vi "Error Process.vi"(8 "error in (no error)":errorcluster, 11 "View Model":T1) -> (0 "error out":errorcluster)   [LabVIEW 2017]
doc: "The Elevator has centralized error handling with three categories of errors."
uses:
  View Model/Controls/View Model.ctl
  View Model/Controls/Shared Model.ctl
  Controls/Error Model.ctl
  Controls/Error Event.ctl
  Controls/Error Type.ctl
  Configuration/Controls/Config DB Model.ctl
  Configuration/Controls/Config DB Command.ctl
  Configuration/Controls/Config DB Record.ctl
  Controller/Controls/Controller Model.ctl
  Controller/Controls/Elevator Location.ctl
  Controller/Controls/Elevator Direction Event.ctl
  Controller/Controls/Elevator Direction.ctl
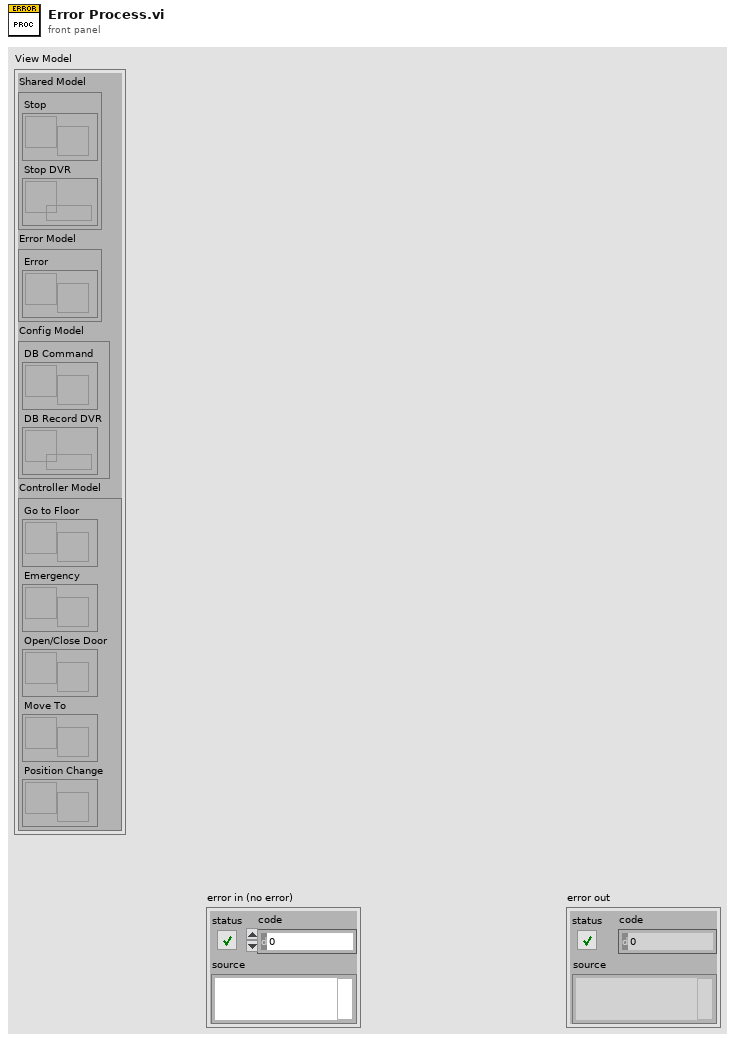
[diagram p1: front panel]
types:
  T1 = typedef "View Model.ctl" = cluster{"Shared Model":T2, "Error Model":T3, "Config Model":T4, "Controller Model":T5}
  T2 = typedef "Shared Model.ctl" = cluster{"Stop":refnum<user-event>, "Stop DVR":refnum<data-value>}
  T3 = typedef "Error Model.ctl" = cluster{"Error":refnum<user-event>}
  T4 = typedef "Config DB Model.ctl" = cluster{"DB Command":refnum<user-event>, "DB Record DVR":refnum<data-value>}
  T5 = typedef "Controller Model.ctl" = cluster{"Go to Floor":refnum<user-event>, "Emergency":refnum<user-event>, "Open/Close Door":refnum<user-event>, "Move To":refnum<user-event>, "Position Change":refnum<user-event>}
  T6 = typedef "Error Type.ctl" = enum16{"Console Error", "Sensor Interface IO Error", "Process Step Error"}
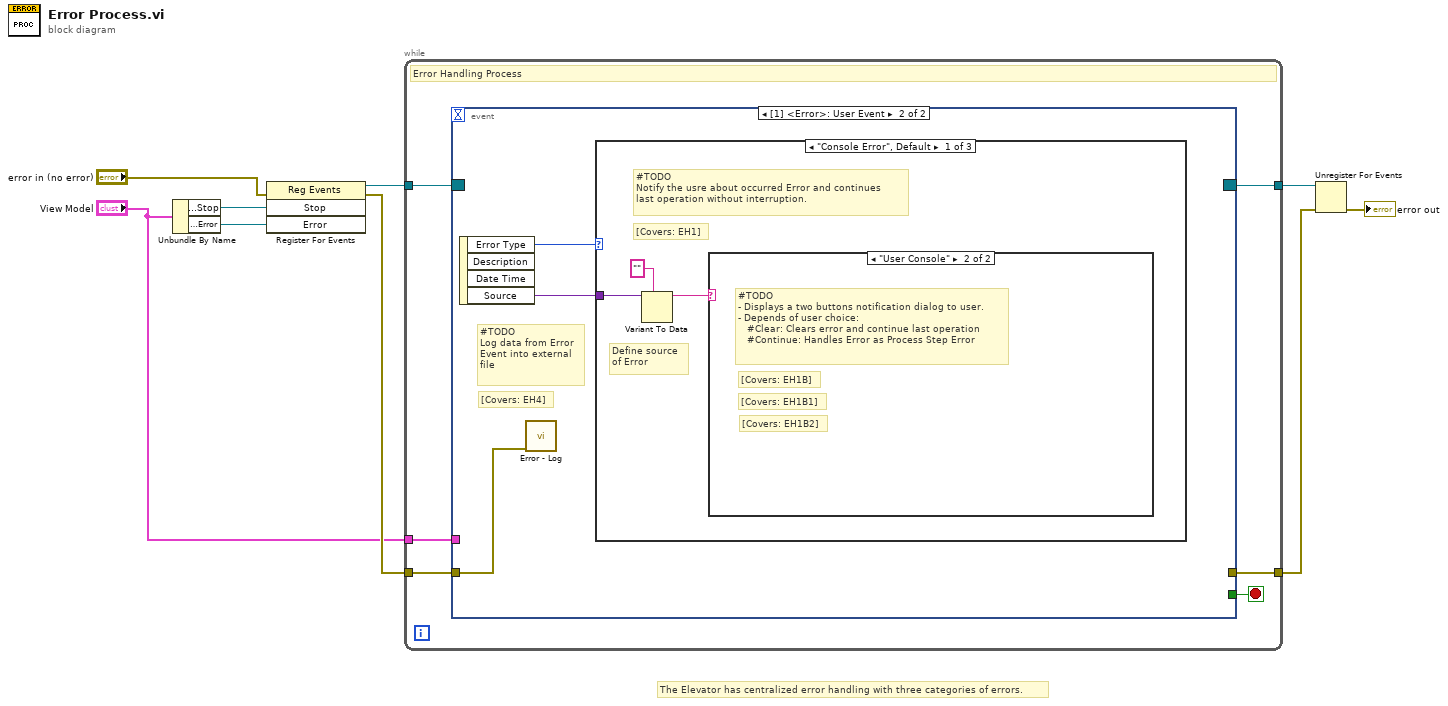
[diagram p0: block diagram]
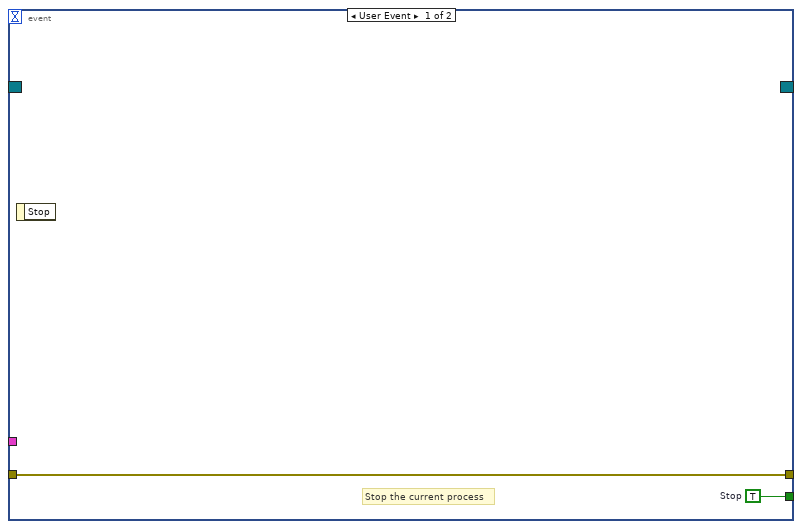
[diagram p2: hidden frame]
diagram:
  # "The Elevator has centralized error handling with three categories of errors."
  n1 = Unbundle By Name("View Model") -> ("Shared Model.Stop"=w9:refnum<user-event>, "Error Model.Error"=w1:refnum<user-event>)
  n2 = register-events(error in="error in (no error)", w9, w1) -> (reference out=w8:refnum<event-registration>, error out=w5:errorcluster)  [unwired: 1 in]
  n3 = while {
    tunnel: w8 -> [w15]
    tunnel: [w14] -> w7
    tunnel: w5 -> [w13]
    tunnel: "View Model" -> [w12]
    tunnel: [w11] -> w3
    stop <- w10 stop-if-true
    # "Error Handling Process"
    n4 = event shown="[1] <Error>: User Event" {
      selector: w15 -> [_ _]
      dyn-events: [_ _] -> w14
      timeout: _ -> [_ _]
      tunnel: w13 -> [w17 w18]
      tunnel: w12 -> [_ _]
      tunnel: [w17 _] -> w11
      tunnel: [w16 _] -> w10
      event User Event {
        w16 = TRUE  # Stop
        # "Stop the current process"
        n5 = event-data() -> ()  [unwired: 1 in, 1 out]
      }
      event User Event {
        # "[Covers: EH4]"
        # "#TODO\nLog data from Error\nEvent into external\nfile"
        n6 = event-data() -> ("Error Type"=w20:T6, "Source"=w19:variant)  [unwired: 1 in, 2 out]
        n7 = call "Error - Log.vi"("error in (no error)"=w18) -> ()  [unwired: 10 in, 1 out]
        n8 = case shown="\"Console Error\", Default" w20 {
          tunnel: w19 -> [w23 _ _]
          frame "Console Error", Default {
            # "Define source \nof Error"
            # "[Covers: EH1]"
            # "#TODO\nNotify the usre about occurred Error and continues \nlast operation without interruption."
            n9 = Variant To Data(type="", Variant=w23) -> (data=w21:string)  [unwired: 1 in, 1 out]
            n10 = case shown="\"User Console\"" w21 {
              frame "Display Console", Default {
                # "[Covers: EH1A]"
                # "#TODO\n- Displays a notification dialog to user.\n- Clears error and continue last operation after dialog is closed."
              }
              frame "User Console" {
                # "[Covers: EH1B2]"
                # "[Covers: EH1B1]"
                # "[Covers: EH1B]"
                # "#TODO\n- Displays a two buttons notification dialog to user.\n- Depends of user choice:\n   #Clear: Clears error and continue last operation\n   #Continue: Handles Error as Process Step Error"
              }
            }
          }
          frame "Sensor Interface IO Error" {
            # "[Covers: EH2]"
            # "#TODO\nTransition to next state = Termination Process"
          }
          frame "Process Step Error" {
            # "[Covers: EH3]"
            # "#TODO\nTransition to next state = Termination Process"
          }
        }
      }
    }
  }
  n11 = Unregister For Events(event registration refnum=w7, error in=w3) -> (error out=→"error out":errorcluster)
